vi "xPCScGetTime.vi"(3 "error in (no error)":errorcluster, 4 "scope":i32, 5 "port":i32) -> (0 "error out":errorcluster, 1 "scope time":dbl format="%.2f", 2 "port copy":i32)   [LabVIEW 2018]
uses:
  XPCAPI.DLL
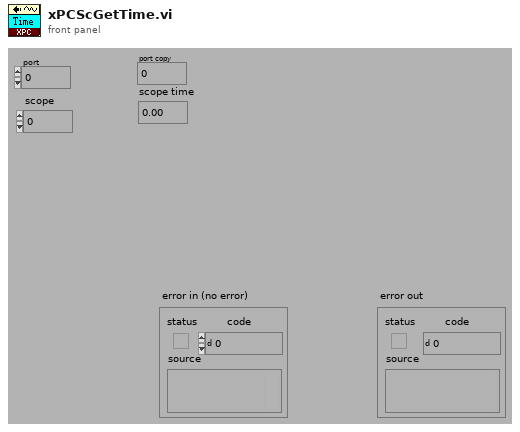
[diagram p1: front panel]
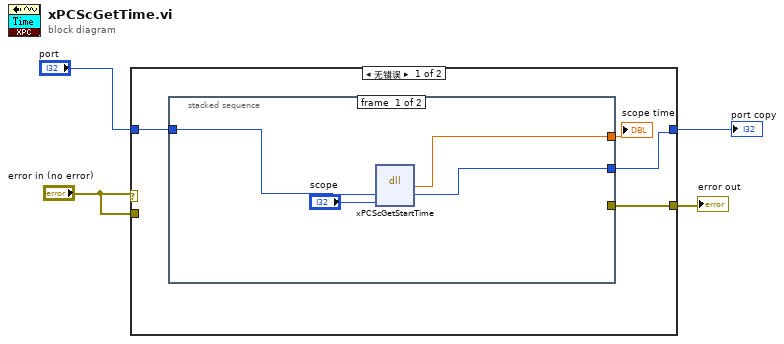
[diagram p0: block diagram]
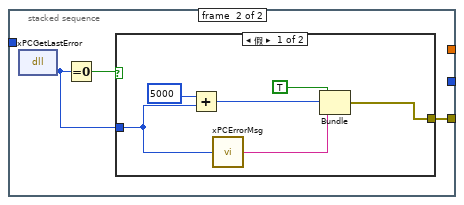
[diagram p2: hidden frame]
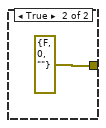
[diagram p3: hidden frame]
diagram:
  n1 = case shown="无错误" "error in (no error)" {
    tunnel: [w8 w24] -> w4
    tunnel: "error in (no error)" -> [_ w24]
    tunnel: "port" -> [w7 w23]
    tunnel: [w6 w23] -> w1
    frame No Error {
      n2 = stacked-sequence {
        tunnel: [w12 _] -> w6
        tunnel: [_ w13] -> w8
        tunnel: w7 -> [w10 _]
        tunnel: [w9 _] -> w5
        frame #0 {
          n3 = dll-call lib="PTH2Iabs CUsers\nyuchengxinDesktop上下位机联机测试\nxpcapi.dll" fn="xPCScGetStartTime"("port"=w10, "scope"="scope") -> ("return type"=w9:dbl, "port"=w12:i32)  [unwired: 4 in, 2 out]
        }
        frame #1 {
          n4 = dll-call lib="PTH2Iabs CUsers\nyuchengxinDesktop上下位机联机测试\nxpcapi.dll" fn="xPCGetLastError"() -> (w14:i32)  [unwired: 3 in, 2 out]
          n5 = Equal To 0?(x=w14) -> (x = 0?=w15:bool)
          n6 = case shown="假" w15 {
            tunnel: w14 -> [w17 _]
            tunnel: [w18 errorcluster {"status"=FALSE, "code"=0, "source"=""} ("error out")] -> w13
            frame False {
              n7 = Add(x=5000 ("y"), y=w17) -> (x+y=w20:i32)
              n8 = call "xPCErrorMsg.vi"("error number"=w17) -> ("ErrorMsg"=w19:string)
              n9 = Bundle(TRUE, w20, "ErrorMsg"=w19) -> (w18:cluster{bool, i32, "ErrorMsg":string})  [unwired: 1 in]
            }
            frame True {
            }
          }
        }
      }
      "scope time" <- w5
    }
    frame Error {
    }
  }
  "port copy" <- w1
  "error out" <- w4
